vi "get_journey.vi"(0 "HGF_Agent in":refnum<class "MoAgSy_AgentBase.lvclass">, 5 "error in (no error)":errorcluster) -> (14 "HGF_Agent out":refnum<class "MoAgSy_AgentBase.lvclass">, 16 "journey":string[](array[string]), 19 "error out":errorcluster)   [LabVIEW 2009, in "MoAgSy_Base.lvlib" / "MoAgSy_AgentBase.lvclass"]
uses:
  MoAgSy_AgentBase.lvclass
  MoAgSy_AgentBase.lvclass/MoAgSy_AgentBase.ctl
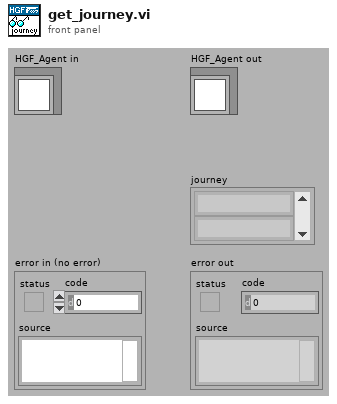
[diagram p1: front panel]
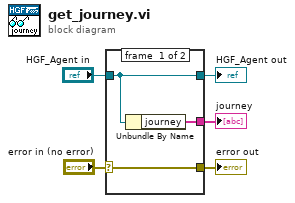
[diagram p0: block diagram]
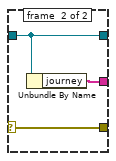
[diagram p2: hidden frame]
diagram:
  n1 = case shown="Error" "error in (no error)" {
    selector: "error in (no error)" -> [w8 w11]
    tunnel: [w8 w11] -> w4
    tunnel: [w7 w10] -> w2
    tunnel: "HGF_Agent in" -> [w7 w10]
    tunnel: [w6 w9] -> w1
    frame #0 {
      n2 = Unbundle By Name(w7) -> ("journey"=w6:string[])
    }
    frame #1 {
      n3 = Unbundle By Name(w10) -> ("journey"=w9:string[])
    }
  }
  "error out" <- w4
  "HGF_Agent out" <- w2
  "journey" <- w1
